vi "Demo_UpdateList.vi"(7 "Offset":i32, 9 "Buffer":T3(array[cluster]) {"Channel" items=["通道1", "通道2"]}, 10 "list":refnum<vi>, 11 "MainVi":refnum<vi>) -> ()   [LabVIEW 2011]
uses:
  ControlCAN/ControlCAN.llb/CAN Channel.ctl
  ControlCAN/ControlCAN.llb/VCI_CAN_OBJ.ctl
  ControlCAN/ControlCAN.lvlib
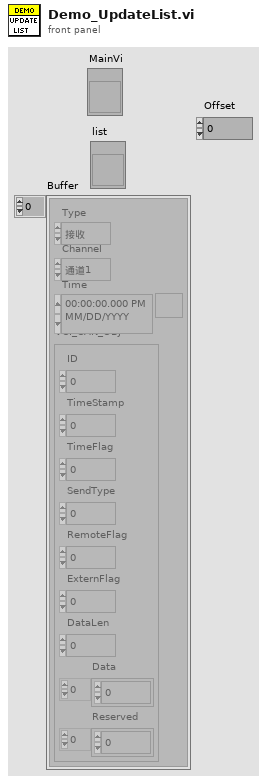
[diagram p1: front panel]
types:
  T1 = typedef "ControlCAN.lvlib/CAN Channel.ctl" = u32
  T2 = typedef "ControlCAN.lvlib/VCI_CAN_OBJ.ctl" = cluster{"ID":u32, "TimeStamp":u32, "TimeFlag":u8, "SendType":u8, "RemoteFlag":u8, "ExternFlag":u8, "DataLen":u8, "Data":u8[], "Reserved":u8[]}
  T3 = cluster{"Type":enum16{"接收", "发送"}, "Channel":T1, "Time":timestamp, "VCI_CAN_OBJ":T2}[]
  T4 = typedef "LVRowAndColumnUnsignedTypeDef.ctl" = cluster{"Row":u32, "Column":u32}
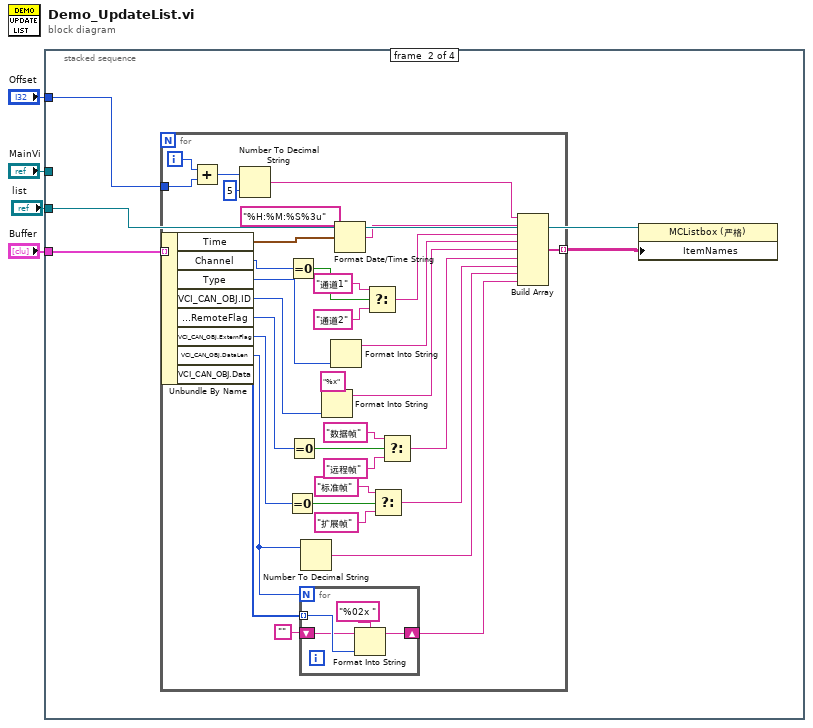
[diagram p0: block diagram]
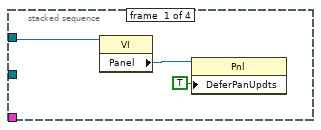
[diagram p2: hidden frame]
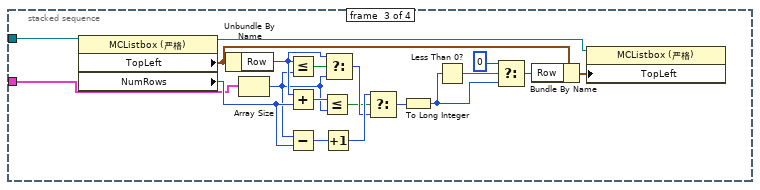
[diagram p3: hidden frame]
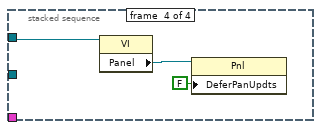
[diagram p4: hidden frame]
diagram:
  n1 = stacked-sequence {
    tunnel: "MainVi" -> [w7 _ _ w72]
    tunnel: "list" -> [_ w8 w53 _]
    tunnel: "Buffer" -> [_ w11 w52 _]
    tunnel: "Offset" -> [_ w10 _ _]
    frame #0 {
      n2 = property class="VI"(reference=w7) -> ("Panel"=w6:refnum<vi>)  [unwired: 1 in, 2 out]
      n3 = property class="Pnl"(reference=w6, "DeferPanUpdts"=TRUE ("延迟前面板更新")) -> ()  [unwired: 1 in, 2 out]
    }
    frame #1 {
      n4 = for {
        tunnel: w11 -> [w42] mode=indexing
        tunnel: w10 -> [w45]
        tunnel: [w12] -> w9 mode=indexing
        i -> [w46]
        n5 = Unbundle By Name(w42) -> ("Time"=w41:timestamp, "Channel"=w39:T1, "Type"=w35:enum16{"接收", "发送"}, "VCI_CAN_OBJ.ID"=w34:u32, "VCI_CAN_OBJ.RemoteFlag"=w32:u8, "VCI_CAN_OBJ.ExternFlag"=w28:u8, "VCI_CAN_OBJ.DataLen"=w24:u8, "VCI_CAN_OBJ.Data"=w23:u8[])
        n6 = Add(x=w46, y=w45) -> (x+y=w44:i32)
        n7 = Number To Decimal String(number=w44, width (-)=i16 5 ("宽度(-)")) -> (decimal integer string=w21:string)
        n8 = Equal To 0?(x=w28) -> (x = 0?=w26:bool)
        n9 = Equal To 0?(x=w39) -> (x = 0?=w38:bool)
        n10 = Equal To 0?(x=w32) -> (x = 0?=w29:bool)
        n11 = for {
          N: w24 -> [_]
          tunnel: w23 -> [w50] mode=indexing
          shift-right: [w47] -> w13
          shift-left: "" -> [w49]
          n12 = Format Into String(format string="%02x " ("格式字符串"), initial string=w49, w50) -> (resulting string=w47:string)  [unwired: 1 in, 1 out]
        }
        n13 = Number To Decimal String(number=w24) -> (decimal integer string=w14:string)  [unwired: 1 out]
        n14 = Format Into String(format string="%x" ("格式字符串"), w34) -> (resulting string=w17:string)  [unwired: 2 in, 1 out]
        n15 = Format Into String(w35) -> (resulting string=w18:string)  [unwired: 3 in, 1 out]
        n16 = Format Date/Time String(time format string (%c)="%H:%M:%S%3u" ("时间格式字符串(%c)"), seconds (now)=w41) -> (date/time string=w20:string)  [unwired: 1 out]
        n17 = Select(t="通道1" ("时间格式字符串(%c)"), s=w38, f="通道2" ("时间格式字符串(%c)")) -> (s? t:f=w19:string)
        n18 = Select(t="标准帧" ("时间格式字符串(%c)"), s=w26, f="扩展帧" ("时间格式字符串(%c)")) -> (s? t:f=w15:string)
        n19 = Select(t="数据帧" ("时间格式字符串(%c)"), s=w29, f="远程帧" ("时间格式字符串(%c)")) -> (s? t:f=w16:string)
        n20 = Build Array(w21, w20, w19, w18, w17, w16, w15, w14, w13) -> (w12:string[])
      }
      n21 = property class="MCListbox (严格)"(reference=w8, "ItemNames"=w9) -> ()  [unwired: 1 in, 2 out]
    }
    frame #2 {
      n22 = property class="MCListbox (严格)"(reference=w53) -> (reference out=w68:refnum<vi>, "TopLeft"=w56:T4, "NumRows"=w55:u32)  [unwired: 1 in, 1 out]
      n23 = Unbundle By Name(w56) -> ("Row"=w58:u32)
      n24 = Array Size(array=w52) -> (size(s)=w51:i32)
      n25 = Less Or Equal?(x=w58, y=w51) -> (x <= y?=w57:bool)
      n26 = Add(x=w58, y=w55) -> (x+y=w59:u32)
      n27 = Subtract(x=w51, y=w55) -> (x-y=w62:u32)
      n28 = Less Or Equal?(x=w59, y=w51) -> (x <= y?=w60:bool)
      n29 = Increment(x=w62) -> (x+1=w63:u32)
      n30 = Select(t=w58, s=w57, f=w51) -> (s? t:f=w61:u32)
      n31 = Select(t=w63, s=w60, f=w61) -> (s? t:f=w64:u32)
      n32 = To Long Integer(number=w64) -> (32bit integer=w66:i32)
      n33 = Less Than 0?(x=w66) -> (x < 0?=w65:bool)
      n34 = Select(t=0, s=w65, f=w66) -> (s? t:f=w54:i32)
      n35 = Bundle By Name(cluster=w56, "Row"=w54) -> (w69:T4)
      n36 = property class="MCListbox (严格)"(reference=w68, "TopLeft"=w69) -> ()  [unwired: 1 in, 2 out]
    }
    frame #3 {
      n37 = property class="VI"(reference=w72) -> ("Panel"=w71:refnum<vi>)  [unwired: 1 in, 2 out]
      n38 = property class="Pnl"(reference=w71, "DeferPanUpdts"=FALSE ("延迟前面板更新")) -> ()  [unwired: 1 in, 2 out]
    }
  }
